vi "GT Open.vi"(8 "error in (no error)":errorcluster caption="错误输入（无错误）", 9 "param":i16, 10 "channel":i16, 11 "cardNum":i16) -> (0 "error out":errorcluster caption="错误输出", 3 "function return":i16)   [LabVIEW 2014, in "gts.lvlib"]
doc: "GT_API GT_Open(short cardNum,short channel=0,short param=1);"
uses:
  gts.lvlib
  gts.dll
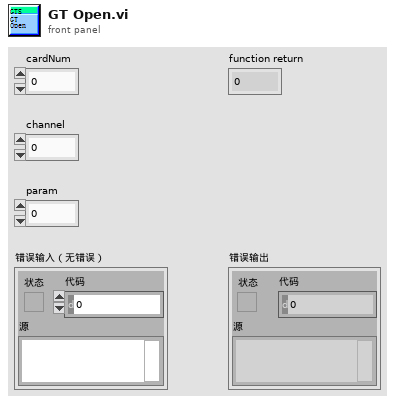
[diagram p1: front panel]
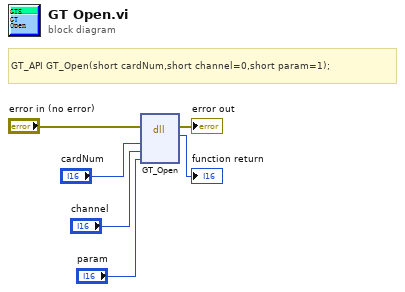
[diagram p0: block diagram]
diagram:
  # "GT_API GT_Open(short cardNum,short channel=0,short param=1);"
  n1 = dll-call lib="PTH2Xabs CUsersgoogolDesktop.多卡库-控制卡基本运动例程(labview)gts.dll" fn="GT_Open"(error in="error in (no error)", "cardNum"="cardNum", "channel"="channel", "param"="param") -> (error out=→"error out":errorcluster, "返回类型"=→"function return":i16)  [unwired: 5 in, 1 out]
